vi "UTILITY Array to String Array.vi"(11 "Hex Array Out":u8[](array[numeric]) format="%x") -> (2 "String":string, 3 "Array":string[](array[string]))   [LabVIEW 2018]
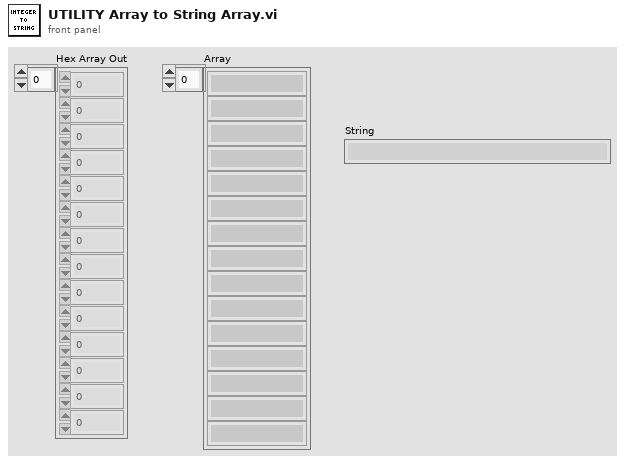
[diagram p1: front panel]
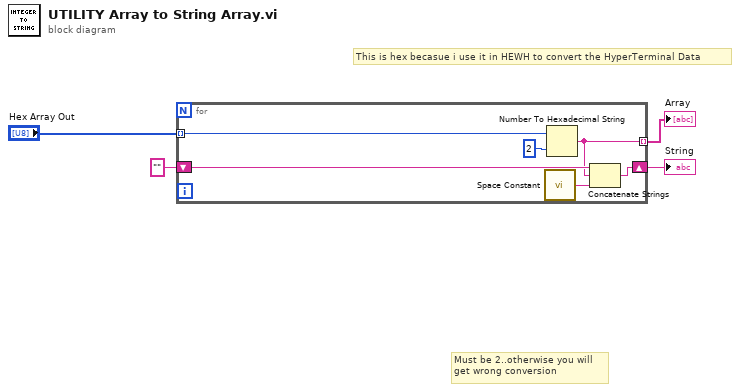
[diagram p0: block diagram]
diagram:
  # "Must be 2..otherwise you will\nget wrong conversion"
  # "This is hex becasue i use it in HEWH to convert the HyperTerminal Data"
  n1 = for {
    tunnel: "Hex Array Out" -> [w10] mode=indexing
    tunnel: [w6] -> w4 mode=indexing
    shift-right: [w7] -> w1
    shift-left: "" -> [w8]
    n2 = call <vilib>:"Space Constant.vi"() -> ("String"=w5:string)
    n3 = Number To Hexadecimal String(1:i16 2 ("width (-)"), 2:w10) -> (0:w6:string)
    n4 = Concatenate Strings(w8, w6, w5) -> (w7:string)
  }
  "Array" <- w4
  "String" <- w1
